vi "Instructor Write Client.vi"() -> ()   [LabVIEW 2017]
uses:
  <vilib>/OPCUA/NI OPC UA Client.lvlib
  <vilib>/OPCUA/controls/Write Status.ctl
  <vilib>/OPCUA/controls/NodeId.ctl
  <vilib>/OPCUA/client/Multiple Write Double Array.vi
panel:
  in  "Stop Broadcasting":bool
  in  "Time Stamp":timestamp
  in  "Node Status":T1 items=["Good"=0, "Uncertain"=1073741824, "Uncertain_InitialValue"=1083310080, "Uncertain_LastUsableValue"=1083179008, "Uncertain_SensorNotAccurate"=1083375616, "Uncertain_EngineeringUnitsExceeded"=1083441152, "Bad"=2147483648, "Bad_NoCommunication"=2150694912, "Bad_NotReadable"=2151284736, "Bad_NotWritable"=2151350272, "Bad_OutOfRange"=2151415808, "Bad_WaitingForInitialData"=2150760448]
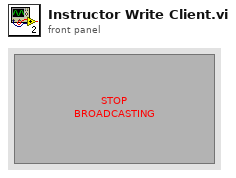
[diagram p1: front panel]
types:
  T1 = typedef "Write Status.ctl" = u32
  T2 = cluster{"message mode":enum16{"None", "Sign", "Sign and Encrypt"}, "security":enum16{"Basic256", "Basic128Rsa15"}}
  T3 = typedef "OPC UA Client Refnum.ctl" = refnum<k21>
  T4 = typedef "NodeId.ctl" = string
  T5 = cluster{"node ID":T4, "value":dbl[], "timestamp (current time)":timestamp, "node status":T1}
  T6 = cluster{"node ID":T4, "value":dbl[], "timestamp (current time)":timestamp, "node status":T1}[]
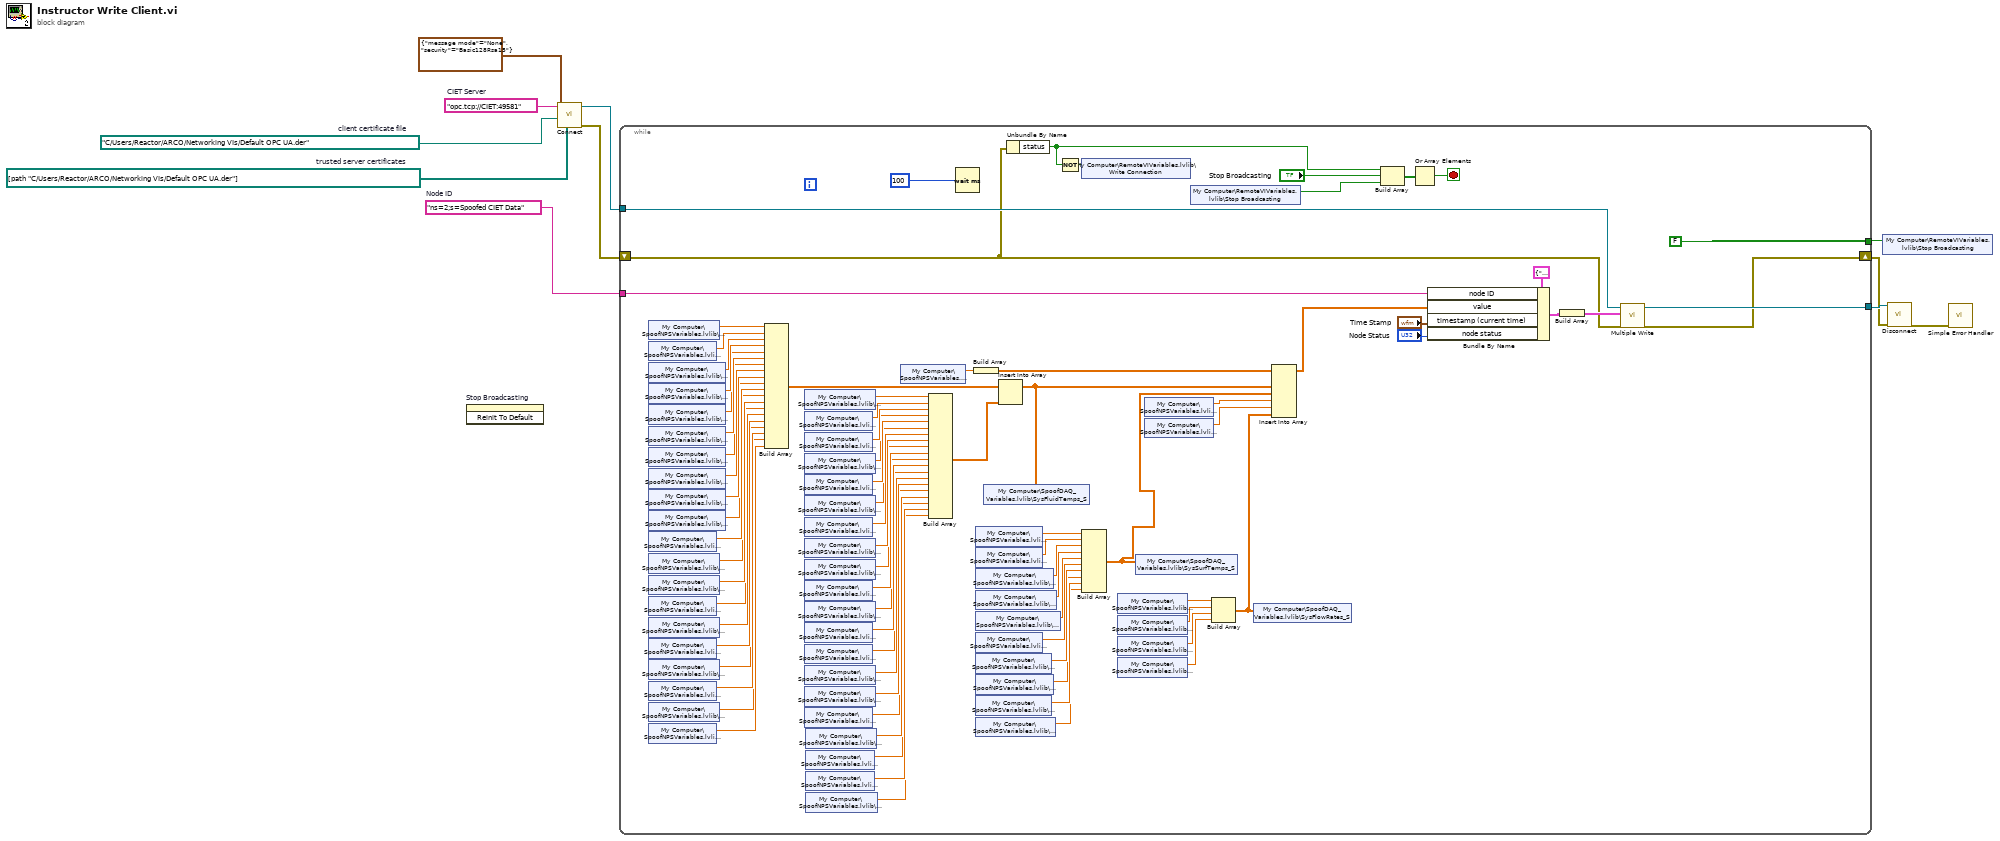
[diagram p0: block diagram]
diagram:
  w5 = path[] [path "C:/Users/Reactor/ARCO/Networking VIs/Default OPC UA.der"]  # trusted server certificates
  w6 = path "C:/Users/Reactor/ARCO/Networking VIs/Default OPC UA.der"  # client certificate file
  w8 = "ns=2;s=Spoofed CIET Data"  # Node ID
  w10 = "opc.tcp://CIET:49581"  # CIET Server
  n1 = invoke on="Stop Broadcasting" class="Bool (strict)" method="Reinit To Default"() -> ()  [unwired: 3 in, 3 out]
  n2 = call <vilib>:"Connect.vi"("trusted server certificates"=w5, "client certificate file"=w6, "security policy"=T2 {"message mode"=enum."None", "security"=enum."Basic128Rsa15"}, "server endpoint URL"=w10) -> ("error out"=w2:errorcluster, "OPC UA client refnum out"=w9:T3)  [unwired: 5 in, 1 out]
  n3 = while {
    tunnel: w8 -> [w92]
    tunnel: w9 -> [w90]
    tunnel: [w91] -> w7
    tunnel: [FALSE] -> w3
    shift-right: [w13] -> w1
    shift-left: w2 -> [w12]
    stop <- w19 stop-if-true
    n4 = shared-variable "My Computer\\SpoofNPSVariables.lvlib\\WT-10_S"() -> (w84:sgl)  [unwired: 1 in, 1 out]
    n5 = shared-variable "My Computer\\SpoofNPSVariables.lvlib\\BT-11_S"() -> (w83:sgl)  [unwired: 1 in, 1 out]
    n6 = shared-variable "My Computer\\SpoofNPSVariables.lvlib\\CX-10-1_S"() -> (w82:sgl)  [unwired: 1 in, 1 out]
    n7 = shared-variable "My Computer\\SpoofNPSVariables.lvlib\\CX-10-2_S"() -> (w81:sgl)  [unwired: 1 in, 1 out]
    n8 = shared-variable "My Computer\\SpoofNPSVariables.lvlib\\CX-10-3_S"() -> (w80:sgl)  [unwired: 1 in, 1 out]
    n9 = shared-variable "My Computer\\SpoofNPSVariables.lvlib\\CX-10-4_S"() -> (w79:sgl)  [unwired: 1 in, 1 out]
    n10 = shared-variable "My Computer\\SpoofNPSVariables.lvlib\\CX-11-1_S"() -> (w78:sgl)  [unwired: 1 in, 1 out]
    n11 = shared-variable "My Computer\\SpoofNPSVariables.lvlib\\CX-11-2_S"() -> (w77:sgl)  [unwired: 1 in, 1 out]
    n12 = shared-variable "My Computer\\SpoofNPSVariables.lvlib\\CX-11-3_S"() -> (w76:sgl)  [unwired: 1 in, 1 out]
    n13 = shared-variable "My Computer\\SpoofNPSVariables.lvlib\\CX-11-4_S"() -> (w75:sgl)  [unwired: 1 in, 1 out]
    n14 = shared-variable "My Computer\\SpoofNPSVariables.lvlib\\BT-12_S"() -> (w74:sgl)  [unwired: 1 in, 1 out]
    n15 = shared-variable "My Computer\\SpoofNPSVariables.lvlib\\WT-13_S"() -> (w73:sgl)  [unwired: 1 in, 1 out]
    n16 = shared-variable "My Computer\\SpoofNPSVariables.lvlib\\WT-20_S"() -> (w72:sgl)  [unwired: 1 in, 1 out]
    n17 = shared-variable "My Computer\\SpoofNPSVariables.lvlib\\BT-21_S"() -> (w71:sgl)  [unwired: 1 in, 1 out]
    n18 = shared-variable "My Computer\\SpoofNPSVariables.lvlib\\WT-22_S"() -> (w70:sgl)  [unwired: 1 in, 1 out]
    n19 = shared-variable "My Computer\\SpoofNPSVariables.lvlib\\BT-23_S"() -> (w69:sgl)  [unwired: 1 in, 1 out]
    n20 = shared-variable "My Computer\\SpoofNPSVariables.lvlib\\WT-24_S"() -> (w68:sgl)  [unwired: 1 in, 1 out]
    n21 = shared-variable "My Computer\\SpoofNPSVariables.lvlib\\BT-25_S"() -> (w67:sgl)  [unwired: 1 in, 1 out]
    n22 = shared-variable "My Computer\\SpoofNPSVariables.lvlib\\WT-26_S"() -> (w66:sgl)  [unwired: 1 in, 1 out]
    n23 = shared-variable "My Computer\\SpoofNPSVariables.lvlib\\BT-27_S"() -> (w65:sgl)  [unwired: 1 in, 1 out]
    n24 = Build Array(w84, w83, w82, w81, w80, w79, w78, w77, w76, w75, w74, w73, w72, w71, w70, w69, w68, w67, w66, w65) -> (w43:sgl[])
    n25 = shared-variable "My Computer\\SpoofNPSVariables.lvlib\\WT-28_S"() -> (w64:sgl)  [unwired: 1 in, 1 out]
    n26 = shared-variable "My Computer\\SpoofNPSVariables.lvlib\\BT-29_S"() -> (w63:sgl)  [unwired: 1 in, 1 out]
    n27 = shared-variable "My Computer\\SpoofNPSVariables.lvlib\\BT-30_S"() -> (w62:sgl)  [unwired: 1 in, 1 out]
    n28 = shared-variable "My Computer\\SpoofNPSVariables.lvlib\\WT-31_S"() -> (w61:sgl)  [unwired: 1 in, 1 out]
    n29 = shared-variable "My Computer\\SpoofNPSVariables.lvlib\\BT-32_S"() -> (w60:sgl)  [unwired: 1 in, 1 out]
    n30 = shared-variable "My Computer\\SpoofNPSVariables.lvlib\\WT-33_S"() -> (w59:sgl)  [unwired: 1 in, 1 out]
    n31 = shared-variable "My Computer\\SpoofNPSVariables.lvlib\\BT-34_S"() -> (w58:sgl)  [unwired: 1 in, 1 out]
    n32 = shared-variable "My Computer\\SpoofNPSVariables.lvlib\\WT-35_S"() -> (w57:sgl)  [unwired: 1 in, 1 out]
    n33 = shared-variable "My Computer\\SpoofNPSVariables.lvlib\\WT-40_S"() -> (w56:sgl)  [unwired: 1 in, 1 out]
    n34 = shared-variable "My Computer\\SpoofNPSVariables.lvlib\\BT-41_S"() -> (w55:sgl)  [unwired: 1 in, 1 out]
    n35 = shared-variable "My Computer\\SpoofNPSVariables.lvlib\\WT-42_S"() -> (w54:sgl)  [unwired: 1 in, 1 out]
    n36 = shared-variable "My Computer\\SpoofNPSVariables.lvlib\\BT-43_S"() -> (w53:sgl)  [unwired: 1 in, 1 out]
    n37 = shared-variable "My Computer\\SpoofNPSVariables.lvlib\\BT-60_S"() -> (w52:sgl)  [unwired: 1 in, 1 out]
    n38 = shared-variable "My Computer\\SpoofNPSVariables.lvlib\\WT-61_S"() -> (w51:sgl)  [unwired: 1 in, 1 out]
    n39 = shared-variable "My Computer\\SpoofNPSVariables.lvlib\\WT-62_S"() -> (w50:sgl)  [unwired: 1 in, 1 out]
    n40 = shared-variable "My Computer\\SpoofNPSVariables.lvlib\\BT-63_S"() -> (w49:sgl)  [unwired: 1 in, 1 out]
    n41 = shared-variable "My Computer\\SpoofNPSVariables.lvlib\\WT-64_S"() -> (w48:sgl)  [unwired: 1 in, 1 out]
    n42 = shared-variable "My Computer\\SpoofNPSVariables.lvlib\\BT-65_S"() -> (w47:sgl)  [unwired: 1 in, 1 out]
    n43 = shared-variable "My Computer\\SpoofNPSVariables.lvlib\\BT-66_S"() -> (w46:sgl)  [unwired: 1 in, 1 out]
    n44 = shared-variable "My Computer\\SpoofNPSVariables.lvlib\\WT-67_S"() -> (w45:sgl)  [unwired: 1 in, 1 out]
    n45 = shared-variable "My Computer\\SpoofNPSVariables.lvlib\\Time_S"() -> (w32:sgl)  [unwired: 1 in, 1 out]
    n46 = Build Array(w64, w63, w62, w61, w60, w59, w58, w57, w56, w55, w54, w53, w52, w51, w50, w49, w48, w47, w46, w45) -> (w44:sgl[])
    n47 = Wait (ms)(milliseconds to wait=u32 100) -> ()  [unwired: 1 out]
    n48 = Build Array(w32) -> (w23:sgl[])
    n49 = shared-variable "My Computer\\SpoofNPSVariables.lvlib\\ST-10_S"() -> (w42:sgl)  [unwired: 1 in, 1 out]
    n50 = shared-variable "My Computer\\SpoofNPSVariables.lvlib\\ST-11_S"() -> (w41:sgl)  [unwired: 1 in, 1 out]
    n51 = shared-variable "My Computer\\SpoofNPSVariables.lvlib\\ST-12-N_S"() -> (w40:sgl)  [unwired: 1 in, 1 out]
    n52 = shared-variable "My Computer\\SpoofNPSVariables.lvlib\\ST-12-SE_S"() -> (w39:sgl)  [unwired: 1 in, 1 out]
    n53 = shared-variable "My Computer\\SpoofNPSVariables.lvlib\\ST-12-SW_S"() -> (w38:sgl)  [unwired: 1 in, 1 out]
    n54 = shared-variable "My Computer\\SpoofNPSVariables.lvlib\\ST-13_S"() -> (w37:sgl)  [unwired: 1 in, 1 out]
    n55 = shared-variable "My Computer\\SpoofNPSVariables.lvlib\\ST-14-E_S"() -> (w36:sgl)  [unwired: 1 in, 1 out]
    n56 = shared-variable "My Computer\\SpoofNPSVariables.lvlib\\ST-14-N_S"() -> (w35:sgl)  [unwired: 1 in, 1 out]
    n57 = shared-variable "My Computer\\SpoofNPSVariables.lvlib\\ST-14-S_S"() -> (w34:sgl)  [unwired: 1 in, 1 out]
    n58 = shared-variable "My Computer\\SpoofNPSVariables.lvlib\\ST-14-W_S"() -> (w33:sgl)  [unwired: 1 in, 1 out]
    n59 = Insert Into Array(array=w43, new element=w44) -> (w31:sgl[])  [unwired: 1 in]
    n60 = shared-variable "My Computer\\SpoofDAQ_Variables.lvlib\\SysFluidTemps_S"(w31) -> ()  [unwired: 1 in, 1 out]
    n61 = Unbundle By Name(w12) -> ("status"=w15:bool)
    n62 = Not(x=w15) -> (.not. x?=w14:bool)
    n63 = shared-variable "My Computer\\RemoteVIVariables.lvlib\\Write Connection"(w14) -> ()  [unwired: 1 in, 1 out]
    n64 = Build Array(w42, w41, w40, w39, w38, w37, w36, w35, w34, w33) -> (w22:sgl[])
    n65 = shared-variable "My Computer\\SpoofNPSVariables.lvlib\\FM-20_S"() -> (w28:sgl)  [unwired: 1 in, 1 out]
    n66 = shared-variable "My Computer\\SpoofNPSVariables.lvlib\\FM-30_S"() -> (w27:sgl)  [unwired: 1 in, 1 out]
    n67 = shared-variable "My Computer\\SpoofNPSVariables.lvlib\\FM-40_S"() -> (w26:sgl)  [unwired: 1 in, 1 out]
    n68 = shared-variable "My Computer\\SpoofNPSVariables.lvlib\\FM-60_S"() -> (w25:sgl)  [unwired: 1 in, 1 out]
    n69 = shared-variable "My Computer\\SpoofDAQ_Variables.lvlib\\SysSurfTemps_S"(w22) -> ()  [unwired: 1 in, 1 out]
    n70 = shared-variable "My Computer\\SpoofNPSVariables.lvlib\\AT-01_S"() -> (w30:sgl)  [unwired: 1 in, 1 out]
    n71 = shared-variable "My Computer\\SpoofNPSVariables.lvlib\\AT-02_S"() -> (w29:sgl)  [unwired: 1 in, 1 out]
    n72 = shared-variable "My Computer\\RemoteVIVariables.lvlib\\Stop Broadcasting"() -> (w17:bool)  [unwired: 1 in, 1 out]
    n73 = Build Array(w28, w27, w26, w25) -> (w24:sgl[])
    n74 = shared-variable "My Computer\\SpoofDAQ_Variables.lvlib\\SysFlowRates_S"(w24) -> ()  [unwired: 1 in, 1 out]
    n75 = Insert Into Array(array=w23, new element #1=w31, new element #2=w22, new element #3=w30, new element #4=w29, new element #5=w24) -> (w21:sgl[])  [unwired: 1 in]
    n76 = Build Array(w15, "Stop Broadcasting", w17) -> (w18:bool[])
    n77 = Or Array Elements(Boolean array=w18) -> (logical OR=w19:bool)
    n78 = Bundle By Name(cluster=T5 {"node ID"="", "value"=[], "timestamp (current time)"=timestamp(0 s since 1904-01-01), "node status"=0} ("request"), "node ID"=w92, "value"=w21, "timestamp (current time)"="Time Stamp", "node status"="Node Status") -> (w86:T5)
    n79 = Build Array(w86) -> (w85:T6)
    n80 = call-poly <vilib>:"Multiple Write.vi"("error in (no error)"=w12, "requests"=w85, "OPC UA client refnum in"=w90) -> ("error out"=w13:errorcluster, "OPC UA client refnum out"=w91:T3)  [unwired: 5 in, 2 out]
  }
  n81 = shared-variable "My Computer\\RemoteVIVariables.lvlib\\Stop Broadcasting"(w3) -> ()  [unwired: 1 in, 1 out]
  n82 = call <vilib>:"Disconnect.vi"("error in (no error)"=w1, "OPC UA client refnum in"=w7) -> ("error out"=w11:errorcluster)  [unwired: 9 in]
  n83 = call <vilib>:"Simple Error Handler.vi"("error in (no error)"=w11) -> ()  [unwired: 4 in, 5 out]
